vi "cv_06-02.vi"() -> ()   [LabVIEW 2013]
panel:
  out "Temperature":cluster{dbl, "Temperature History":dbl}(graph)
  in  "Power":bool
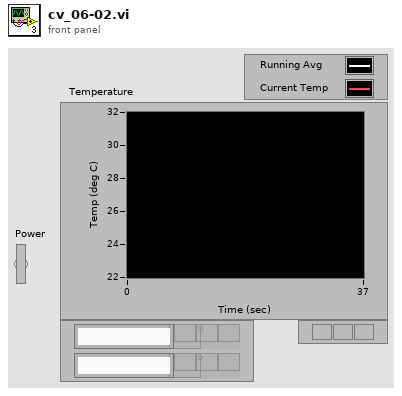
[diagram p1: front panel]
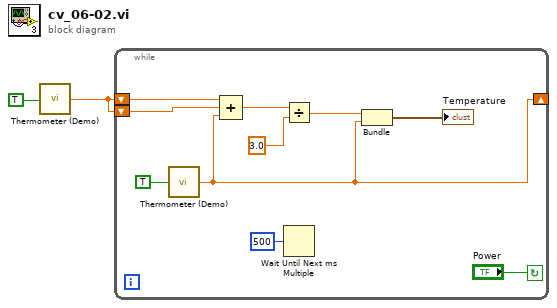
[diagram p0: block diagram]
diagram:
  n1 = call "Thermometer (Demo).vi"("Temp Scale"=TRUE) -> ("Temperature"=w2:dbl)
  n2 = while {
    shift-right: [w4] -> _
    shift-left: w2 -> [w11]
    shift-left: w2 -> [w10]
    stop <- "Power" continue-if-true
    n3 = call "Thermometer (Demo).vi"("Temp Scale"=TRUE) -> ("Temperature"=w4:dbl)
    n4 = Compound Arithmetic op=ADD(w11, w10, w4) -> (w9:dbl)
    n5 = Divide(x=w9, y=3.0) -> (x/y=w6:dbl)
    n6 = Wait Until Next ms Multiple(millisecond multiple=500) -> ()  [unwired: 1 out]
    n7 = Bundle(w6, "Temperature"=w4) -> (→"Temperature":cluster{dbl, "Temperature":dbl})  [unwired: 1 in]
  }
